vi "com接收.vi"(8 "接收数据长度":i32, 10 "RS232波特率":T1(ring), 11 "COM端口":refnum<visa-resource-name>="COM1") -> (0 "超时?":bool, 3 "匹配字符串":string)   [LabVIEW 2010]
uses:
  <vilib>/Instr/_visa.llb/VISA Configure Serial Port (Instr).vi
panel:
  out "Read String":string
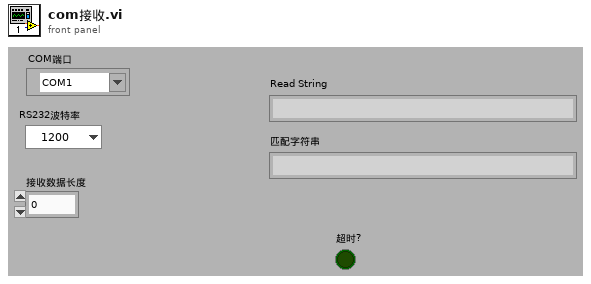
[diagram p1: front panel]
types:
  T1 = enum16{"1200", "2400", "4800", "9600", "19200", "57600", "115200", ""}
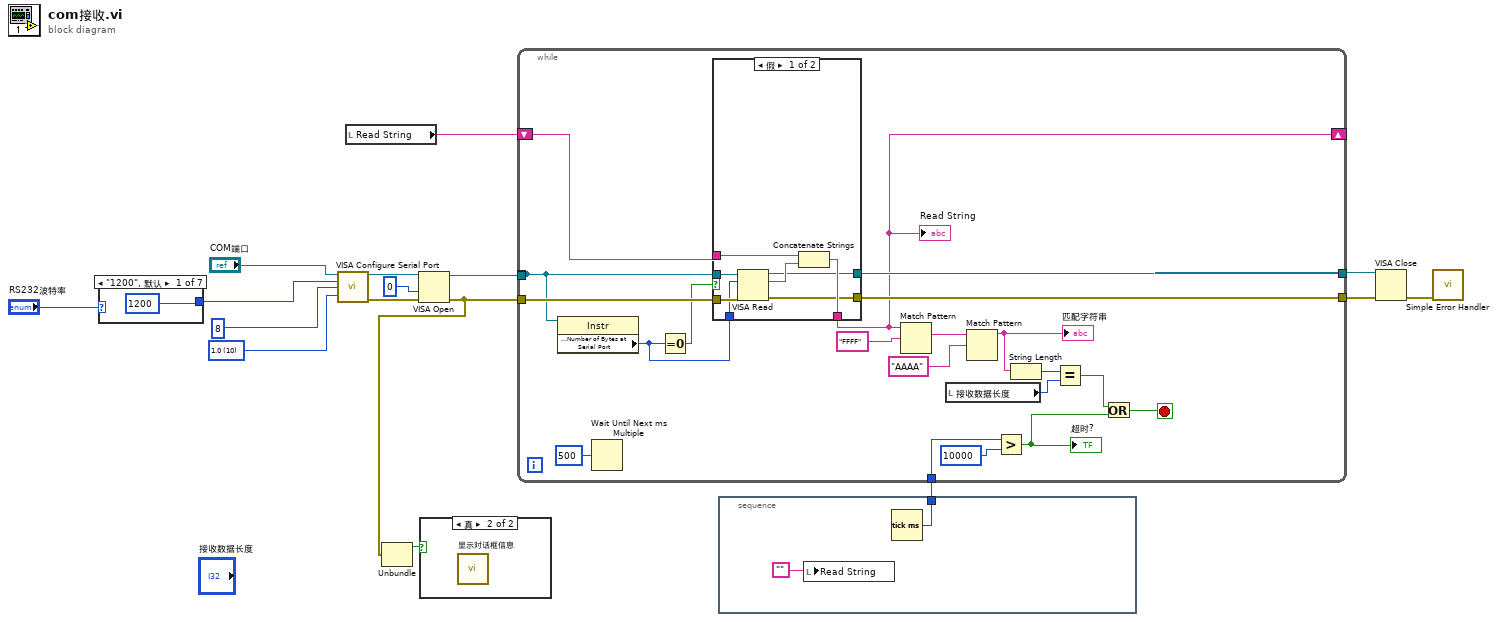
[diagram p0: block diagram]
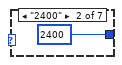
[diagram p2: hidden frame]
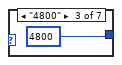
[diagram p3: hidden frame]
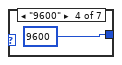
[diagram p4: hidden frame]
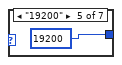
[diagram p5: hidden frame]
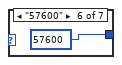
[diagram p6: hidden frame]
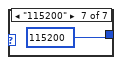
[diagram p7: hidden frame]
diagram:
  w7 = u16 10 items=["1.0"=10, "1.5"=15, "2.0"=20] ("stop bits (10: 1 bit)")
  n1 = case shown="\"1200\", 默认" "RS232波特率" {
    tunnel: [u32 1200 u32 2400 u32 4800 u32 9600 u32 19200 u32 57600 u32 115200] -> w3
    frame "1200", Default {
    }
    frame "2400" {
    }
    frame "4800" {
    }
    frame "9600" {
    }
    frame "19200" {
    }
    frame "57600" {
    }
    frame "115200" {
    }
  }
  n2 = call-poly "VISA Configure Serial Port"("VISA resource name"="COM端口", "baud rate (9600)"=w3, "data bits (8)"=u16 8, "stop bits (10: 1 bit)"=w7) -> ("VISA resource name out"=w13:refnum<visa-resource-name>, "error out"=w9:errorcluster)  [unwired: 10 in]
  n3 = local read "Read String"() -> (w5:string)
  n4 = VISA Open(access mode=u32 0, error in (no error)=w9, VISA resource name=w13) -> (VISA resource name=w12:refnum<visa-resource-name>, error out=w6:errorcluster)  [unwired: 2 in]
  n5 = Unbundle(w6) -> ("status"=w8:bool)  [unwired: 2 out]
  n6 = case shown="真" w8 {
    frame False {
    }
    frame True {
      n7 = call "显示对话框信息"() -> ()  [unwired: 10 in, 2 out]
    }
  }
  n8 = stacked-sequence {
    tunnel: [w24] -> w1
    frame #0 {
      n9 = local write "Read String"("") -> ()
      n10 = Tick Count (ms)() -> (millisecond timer value=w24:u32)
    }
  }
  n11 = while {
    tunnel: [w41] -> _
    tunnel: w6 -> [w45]
    shift-right: [w26] -> _
    shift-left: w5 -> [w44]
    tunnel: [w43] -> w16
    tunnel: [w42] -> w15
    tunnel: w12 -> [w41]
    tunnel: w1 -> [w34]
    stop <- w35 stop-if-true
    n12 = property class="Instr"(reference=w41) -> ("Serial Settings:Number of Bytes at Serial Port"=w39:u32)  [unwired: 1 in, 2 out]
    n13 = Wait Until Next ms Multiple(millisecond multiple=u32 500 ("毫秒倍数")) -> ()  [unwired: 1 out]
    n14 = Equal To 0?(x=w39) -> (x = 0?=w40:bool)
    n15 = case shown="假" w40 {
      tunnel: w45 -> [w53 w55]
      tunnel: [w52 w54] -> w26
      tunnel: w44 -> [w51 w54]
      tunnel: [w49 w56] -> w43
      tunnel: [w48 w55] -> w42
      tunnel: w41 -> [w47 w56]
      tunnel: w39 -> [w46 _]
      frame False {
        n16 = VISA Read(VISA resource name=w47, byte count=w46, error in (no error)=w53) -> (VISA resource name out=w49:refnum<visa-resource-name>, read buffer=w50:string, error out=w48:errorcluster)  [unwired: 1 out]
        n17 = Concatenate Strings(w51, w50) -> (w52:string)
      }
      frame True {
      }
    }
    "Read String" <- w26
    n18 = Match Pattern(string=w26, regular expression="FFFF" ("正则表达式")) -> (match substring=w30:string)  [unwired: 1 in, 3 out]
    n19 = local read "接收数据长度"() -> (w37:i32)
    n20 = Match Pattern(string=w30, regular expression="AAAA" ("正则表达式")) -> (before substring=w28:string)  [unwired: 1 in, 3 out]
    "匹配字符串" <- w28
    n21 = Greater?(x=w34, y=u32 10000) -> (0:w32:bool)
    "超时?" <- w32
    n22 = String Length(string=w28) -> (length=w38:i32)
    n23 = Equal?(x=w38, y=w37) -> (x = y?=w27:bool)
    n24 = Or(x=w27, y=w32) -> (x .or. y?=w35:bool)
  }
  n25 = VISA Close(VISA resource name=w16, error in (no error)=w15) -> (error out=w14:errorcluster)
  n26 = call <vilib>:"Simple Error Handler.vi"("error in (no error)"=w14) -> ()  [unwired: 4 in, 5 out]
